vi "Mode Code 16 with Start Stop and Status.vi"(7 "base name for channel aliases":string, 8 "error in":errorcluster, 11 "Loopback in":refnum<class "Loopback.lvclass">) -> (0 "error out":errorcluster, 3 "Loopback out":refnum<class "Loopback.lvclass">)   [LabVIEW 2020, in "Loopback.lvclass"]
uses:
  Loopback.lvclass
  C:/Git/niveristand-custom-device-testing-tools/VeriStandTestCase/VeriStandTestCase.lvclass
  <vilib>/numeric/Random Number (Range) U64.vi
  a677bd6a-3f62-4bdd-a7cf-3a1725f4fe5c.vi
  <vilib>/numeric/sub_Random U32.vi
  <vilib>/NI VeriStand/Execution/Workspace/NI VeriStand - Set Single Channel Value.vi
  <vilib>/NI VeriStand/Execution/Workspace/NI VeriStand - Get Multiple Channel Values.vi
  <vilib>/NI VeriStand/Execution/Workspace/NI_VS Workspace ExecutionAPI.lvlib
  niveristand-custom-device-testing-tools/VeriStandTestUtilities/VeriStandTestUtilities.lvlib
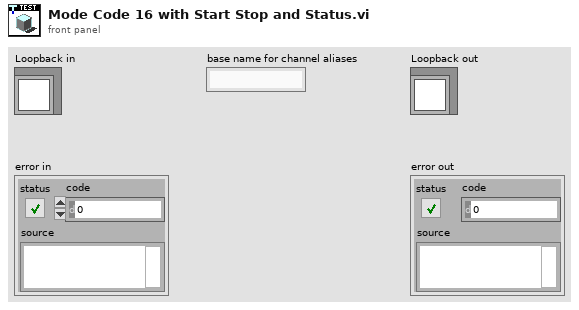
[diagram p1: front panel]
types:
  T1 = typedef "NI_VS Workspace ExecutionAPI.lvlib/WorkspaceAPI.ctl" = refnum<k24>
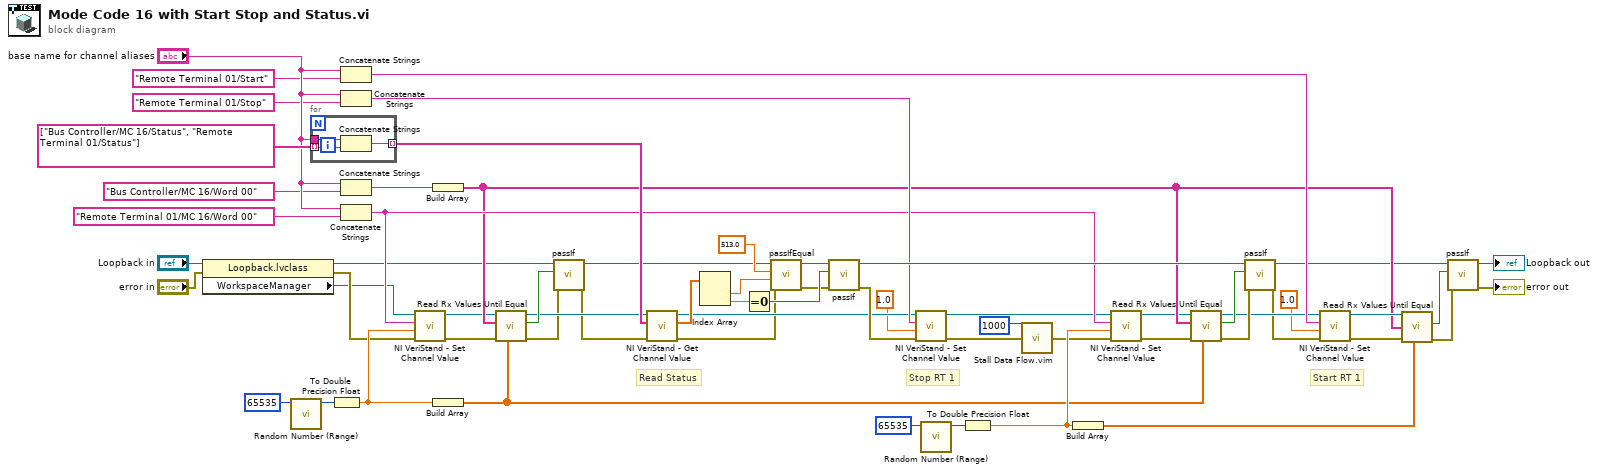
[diagram p0: block diagram]
diagram:
  # "Read Status"
  # "Start RT 1"
  # "Stop RT 1"
  n1 = property class="Loopback.lvclass"(reference="Loopback in", error in="error in") -> (reference out=w2:refnum<class "Loopback.lvclass">, error out=w3:errorcluster, "WorkspaceManager"=w1:T1)
  n2 = call-poly <vilib>:"Random Number (Range).vi"("upper bound (100)"=u64 65535) -> ("number"=w6:u64)  [unwired: 10 in]
  n3 = for {
    tunnel: string[] ["Bus Controller/MC 16/Status", "Remote Terminal 01/Status"] -> [w65] mode=indexing
    tunnel: "base name for channel aliases" -> [w64]
    tunnel: [w63] -> w54 mode=indexing
    n4 = Concatenate Strings(w64, w65) -> (w63:string)
  }
  n5 = To Double Precision Float(number=w6) -> (double precision float=w23:dbl)
  n6 = Concatenate Strings("base name for channel aliases", "Remote Terminal 01/Start" ("Channel")) -> (w49:string)
  n7 = Concatenate Strings("base name for channel aliases", "Remote Terminal 01/Stop" ("Channel")) -> (w51:string)
  n8 = Concatenate Strings("base name for channel aliases", "Bus Controller/MC 16/Word 00" ("Channel")) -> (w45:string)
  n9 = Concatenate Strings("base name for channel aliases", "Remote Terminal 01/MC 16/Word 00" ("Channel")) -> (w47:string)
  n10 = call-poly <vilib>:"NI VeriStand - Set Channel Value.vi"("error in (no error)"=w3, "Value"=w23, "Channel"=w47, "WorkspaceManager in"=w1) -> ("error out"=w25:errorcluster, "WorkspaceManager out"=w24:T1)  [unwired: 6 in]
  n11 = Build Array(w45) -> (w35:string[])
  n12 = Build Array(w23) -> (w31:dbl[])
  n13 = call "Read Rx Values Until Equal.vi"("expected values"=w31, "error in"=w25, "Rx aliases"=w35, "workspace manager in"=w24) -> ("error out"=w26:errorcluster, "values equal expected"=w28:bool, "workspace manager out"=w27:T1)  [unwired: 5 in]
  n14 = call-dynamic "passIf.vi"("error in (no error)"=w26, "pass"=w28, "TestCase in"=w2) -> ("error out"=w19:errorcluster, "TestCase out"=w20:refnum<class "Loopback.lvclass">)  [unwired: 7 in]
  n15 = call-poly <vilib>:"NI VeriStand - Get Channel Value.vi"("error in (no error)"=w19, "Channels"=w54, "WorkspaceManager in"=w27) -> ("error out"=w18:errorcluster, "Values"=w22:dbl[], "WorkspaceManager out"=w21:T1)  [unwired: 6 in]
  n16 = Index Array(array=w22) -> (element #1=w56:dbl, element #2=w55:dbl)  [unwired: 2 in]
  n17 = Equal To 0?(x=w55) -> (x = 0?=w61:bool)
  n18 = call-dynamic "passIfEqual.vi"("error in (no error)"=w18, "y"=w56, "x"=513.0 ("element"), "TestCase in"=w20) -> ("error out"=w57:errorcluster, "TestCase out"=w59:refnum<class "Loopback.lvclass">)  [unwired: 6 in]
  n19 = call-dynamic "passIf.vi"("error in (no error)"=w57, "pass"=w61, "TestCase in"=w59) -> ("error out"=w58:errorcluster, "TestCase out"=w60:refnum<class "Loopback.lvclass">)  [unwired: 7 in]
  n20 = call-poly <vilib>:"NI VeriStand - Set Channel Value.vi"("error in (no error)"=w58, "Value"=1.0, "Channel"=w51, "WorkspaceManager in"=w21) -> ("error out"=w9:errorcluster, "WorkspaceManager out"=w12:T1)  [unwired: 6 in]
  n21 = call-poly <vilib>:"Random Number (Range).vi"("upper bound (100)"=u64 65535) -> ("number"=w14:u64)  [unwired: 10 in]
  n22 = To Double Precision Float(number=w14) -> (double precision float=w40:dbl)
  n23 = call "Stall Data Flow.vim"("value in"=w9, "milliseconds to wait"=u32 1000) -> ("value out"=w11:errorcluster)  [unwired: 1 out]
  n24 = Build Array(w40) -> (w38:dbl[])
  n25 = call-poly <vilib>:"NI VeriStand - Set Channel Value.vi"("error in (no error)"=w11, "Value"=w40, "Channel"=w47, "WorkspaceManager in"=w12) -> ("error out"=w30:errorcluster, "WorkspaceManager out"=w29:T1)  [unwired: 6 in]
  n26 = call "Read Rx Values Until Equal.vi"("expected values"=w31, "error in"=w30, "Rx aliases"=w35, "workspace manager in"=w29) -> ("error out"=w33:errorcluster, "values equal expected"=w34:bool, "workspace manager out"=w32:T1)  [unwired: 5 in]
  n27 = call-dynamic "passIf.vi"("error in (no error)"=w33, "pass"=w34, "TestCase in"=w60) -> ("error out"=w16:errorcluster, "TestCase out"=w17:refnum<class "Loopback.lvclass">)  [unwired: 7 in]
  n28 = call-poly <vilib>:"NI VeriStand - Set Channel Value.vi"("error in (no error)"=w16, "Value"=1.0, "Channel"=w49, "WorkspaceManager in"=w32) -> ("error out"=w37:errorcluster, "WorkspaceManager out"=w36:T1)  [unwired: 6 in]
  n29 = call "Read Rx Values Until Equal.vi"("expected values"=w38, "error in"=w37, "Rx aliases"=w35, "workspace manager in"=w36) -> ("error out"=w39:errorcluster, "values equal expected"=w41:bool)  [unwired: 5 in, 1 out]
  n30 = call-dynamic "passIf.vi"("error in (no error)"=w39, "pass"=w41, "TestCase in"=w17) -> ("error out"=→"error out":errorcluster, "TestCase out"=→"Loopback out":refnum<class "Loopback.lvclass">)  [unwired: 7 in]
